vi "error_display.vi"(6 "NG_add":string, 7 "OK_add":string, 8 "error in":errorcluster, 9 "Action name":string, 10 "return":i32, 11 "DLL path":path) -> (0 "error out":errorcluster, 3 "路径输出":path)   [LabVIEW 2014]
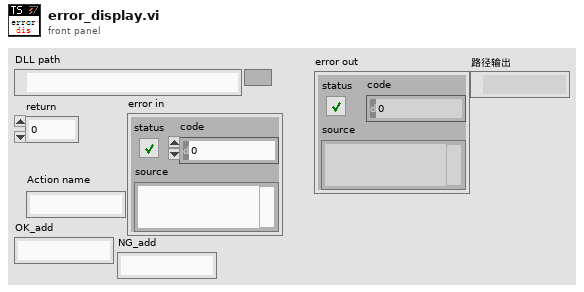
[diagram p1: front panel]
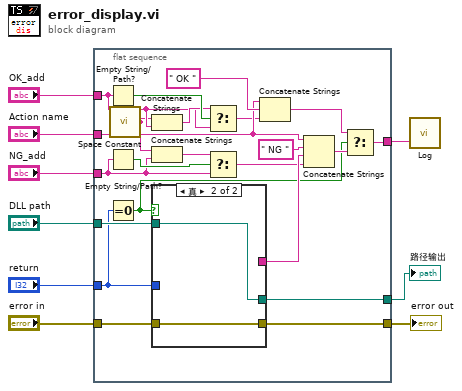
[diagram p0: block diagram]
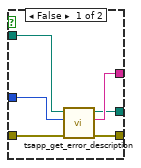
[diagram p2: hidden frame]
diagram:
  n1 = flat-sequence {
    tunnel: [w28] -> w9
    tunnel: "DLL path" -> [w26]
    tunnel: "return" -> [w25]
    tunnel: "Action name" -> [w23]
    tunnel: "error in" -> [w22]
    tunnel: [w21] -> w4
    tunnel: [w20] -> w3
    tunnel: "OK_add" -> [w14]
    tunnel: "NG_add" -> [w12]
    frame #0 {
      n2 = Empty String/Path?(string/path=w14) -> (empty?=w19:bool)
      n3 = Empty String/Path?(string/path=w12) -> (empty?=w15:bool)
      n4 = Equal To 0?(x=w25) -> (x = 0?=w10:bool)
      n5 = call <vilib>:"Space Constant.vi"() -> ("String"=w13:string)
      n6 = Concatenate Strings(w13, w14) -> (w18:string)
      n7 = Concatenate Strings(w13, w12) -> (w16:string)
      n8 = case shown="真" w10 {
        tunnel: [w37 _] -> w27
        tunnel: w26 -> [w36 w39]
        tunnel: w25 -> [w35 _]
        tunnel: w22 -> [w34 w38]
        tunnel: [w33 w38] -> w21
        tunnel: [w32 w39] -> w20
        frame False {
          n9 = call "tsapp_get_error_description.vi"("error in"=w34, "ACount"=w35, "路径输入"=w36) -> ("error out"=w33:errorcluster, "ErrDes"=w37:string, "路径输出"=w32:path)  [unwired: 6 in]
        }
        frame True {
        }
      }
      n10 = Select(t=w18, s=w19, f=w14) -> (s? t:f=w17:string)
      n11 = Select(t=w16, s=w15, f=w12) -> (s? t:f=w11:string)
      n12 = Concatenate Strings(w23, " OK ", w17) -> (w24:string)
      n13 = Concatenate Strings(w23, " NG ", w27, w11) -> (w30:string)
      n14 = Select(t=w24, s=w10, f=w30) -> (s? t:f=w28:string)
    }
  }
  n15 = call "Log.vi"("Data"=w9) -> ()  [unwired: 3 in]
  "error out" <- w4
  "路径输出" <- w3
